vi "E4_Error in_Out.vi"() -> ()   [LabVIEW 2020]
panel:
  out "Square root":dbl
  out "error out":errorcluster
  in  "error in (no error)":errorcluster
  in  "Number":dbl
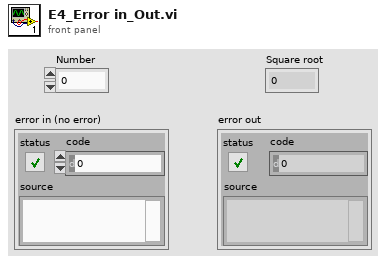
[diagram p1: front panel]
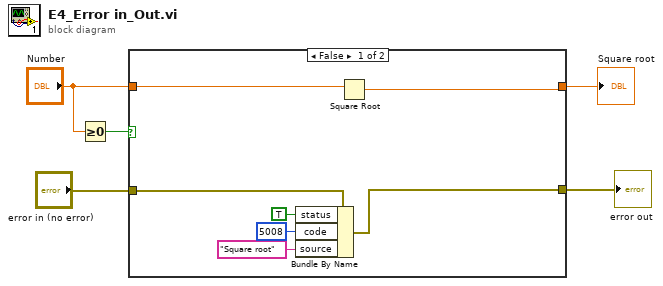
[diagram p0: block diagram]
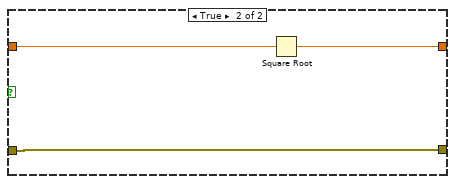
[diagram p2: hidden frame]
diagram:
  n1 = Greater Or Equal To 0?(x="Number") -> (x >= 0?=w5:bool)
  n2 = case shown="False" w5 {
    tunnel: "Number" -> [w7 w14]
    tunnel: "error in (no error)" -> [w12 w15]
    tunnel: [w11 w15] -> w2
    tunnel: [w6 w13] -> w1
    frame False {
      n3 = Bundle By Name(cluster=w12, "status"=TRUE, "code"=5008, "source"="Square root") -> (w11:errorcluster)
      n4 = Square Root(x=w7) -> (sqrt(x)=w6:dbl)
    }
    frame True {
      n5 = Square Root(x=w14) -> (sqrt(x)=w13:dbl)
    }
  }
  "error out" <- w2
  "Square root" <- w1
